vi "ReportMeas.vi"(6 "addr/port":cluster{"address":string, "port":i32}={"address"="127.0.0.1", "port"=31415}, 8 "error in (no error)":errorcluster, 9 "s":dbl, 10 "y":dbl, 11 "x":dbl) -> (0 "error out":errorcluster, 3 "reply out":string)   [LabVIEW 2015]
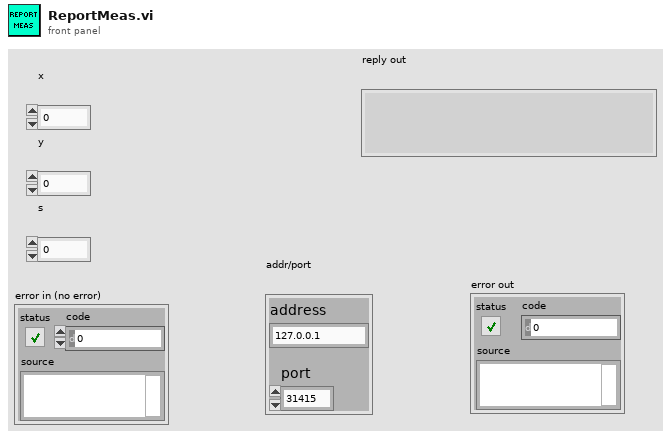
[diagram p1: front panel]
types:
  T1 = cluster{"command":string, "x":dbl, "y":dbl, "s":dbl}
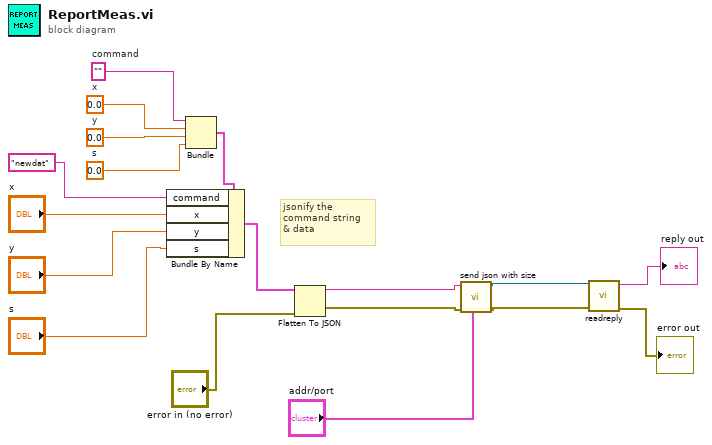
[diagram p0: block diagram]
diagram:
  w2 = 0.0  # s
  w13 = 0.0  # y
  w16 = 0.0  # x
  w17 = ""  # command
  # "jsonify the \ncommand string \n& data"
  n1 = Bundle("command"=w17, "x"=w16, "y"=w13, "s"=w2) -> (w15:T1)  [unwired: 1 in]
  n2 = Bundle By Name(cluster=w15, "command"="newdat", "x"="x", "y"="y", "s"="s") -> (w14:T1)
  n3 = Flatten To JSON(anything=w14, error in (no error)="error in (no error)") -> (JSON string=w3:string, 11:w4:errorcluster)  [unwired: 1 in]
  n4 = call "send json with size.vi"("addr/port"="addr/port", "error in"=w4, "json string"=w3) -> ("error out"=w6:errorcluster, "connection ID out"=w7:refnum<k5>)  [unwired: 6 in, 1 out]
  n5 = call "readreply.vi"("error in (no error)"=w6, "connection ID"=w7) -> ("error out"=→"error out":errorcluster, "data out"=→"reply out":string)  [unwired: 8 in]
